vi "Detect CMD Change.vi"(10 "CMD_ACT_SwerveDrive_Data":T1 {"Auto Angle" scale format="%.3f"; "Direction"."Rotate(Yaw) CCW 1 CW -1" scale=1.0..-1.0; "Direction"."Traverse"."Angle" scale format="%.3f"; "Direction"."Traverse"."Velocity" scale=-1.0..1.0 scale format="%.1f"}, 11 "Preious ACT Input":T1 {"Auto Angle" scale format="%.3f"; "Direction"."Rotate(Yaw) CCW 1 CW -1" scale=1.0..-1.0; "Direction"."Traverse"."Angle" scale format="%.3f"; "Direction"."Traverse"."Velocity" scale=-1.0..1.0 scale format="%.1f"}) -> (3 "New Command":bool)   [LabVIEW 2023, in "Thor-SwerveDrive_ACT.lvlib"]
uses:
  Thor-SwerveDrive_ACT.lvlib
  Shared Code/TypeDefs/ENUM_Swerve_CMD_Mode Select.ctl
  Shared Code/TypeDefs/Level_Velocity plus-minus 1.ctl
  Shared Code/TypeDefs/Dial_Compase heading unit circle CCW positive.ctl
  Shared Code/TypeDefs/Cluster_Module Velocity-Direction-Rotations.ctl
  Type Defs/NUM_Rotate Input.ctl
  Shared Code/TypeDefs/Cluster_CMD_Direction Data.ctl
  Shared Code/TypeDefs/Cluster_X-Y.ctl
  Cluster_CMD_ACT_Data.ctl
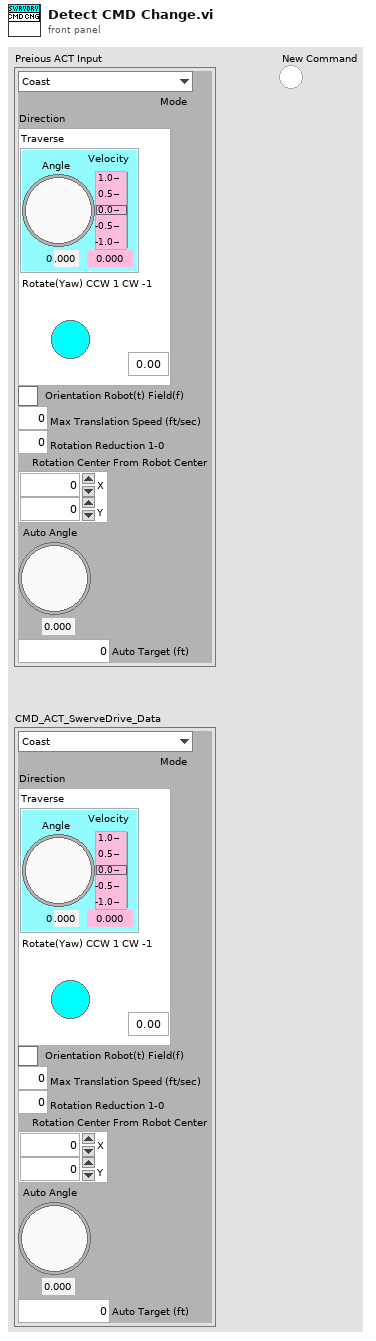
[diagram p1: front panel]
types:
  T1 = typedef "Thor-SwerveDrive_ACT.lvlib/Cluster_CMD_ACT_Data.ctl" = cluster{"Mode":T2, "Direction":T3, "Orientation Robot(t) Field(f)":bool, "Max Translation Speed (ft/sec)":dbl, "Rotation Reduction 1-0":dbl, "Rotation Center From Robot Center":T8, "Auto Angle":T6, "Auto Target (ft)":dbl}
  T2 = typedef "ENUM_Swerve_CMD_Mode Select.ctl" = enum16{"Coast", "Manual", "Auto Trans Auto Rotate", "Manual Trans Auto Rotate", "Balance", "Stop Brake", "Lock Wheels"}
  T3 = typedef "Cluster_CMD_Direction Data.ctl" = cluster{"Traverse":T4, "Rotate(Yaw) CCW 1 CW -1":T7}
  T4 = typedef "Cluster_Module Velocity-Direction-Rotations.ctl" = cluster{"Velocity":T5, "Angle":T6, "Rotations Count":dbl}
  T5 = typedef "Level_Velocity plus-minus 1.ctl" = dbl
  T6 = typedef "Dial_Compase heading unit circle CCW positive.ctl" = dbl
  T7 = typedef "NUM_Rotate Input.ctl" = dbl
  T8 = typedef "Cluster_X-Y.ctl" = cluster{"X":dbl, "Y":dbl}
  T9 = cluster{"Mode":bool, "Direction":cluster{"Traverse":cluster{"Velocity":bool, "Angle":bool, "Rotations Count":bool}, "Rotate(Yaw) CCW 1 CW -1":bool}, "Orientation Robot(t) Field(f)":bool, "Max Translation Speed (ft/sec)":bool, "Rotation Reduction 1-0":bool, "Rotation Center From Robot Center":cluster{"X":bool, "Y":bool}, "Auto Angle":bool, "Auto Target (ft)":bool}
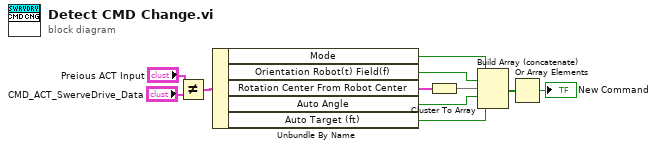
[diagram p0: block diagram]
diagram:
  n1 = Not Equal?(x="Preious ACT Input", y="CMD_ACT_SwerveDrive_Data") -> (x != y?=w9:T9)
  n2 = Unbundle By Name(w9) -> ("Mode"=w5:bool, "Orientation Robot(t) Field(f)"=w6:bool, "Rotation Center From Robot Center"=w8:cluster{"X":bool, "Y":bool}, "Auto Angle"=w4:bool, "Auto Target (ft)"=w3:bool)
  n3 = Cluster To Array(cluster=w8) -> (array=w7:bool[])
  n4 = Build Array (concatenate)(w5, w6, w7, w4, w3) -> (w2:bool[])
  n5 = Or Array Elements(Boolean array=w2) -> (logical OR=→"New Command":bool)
